vi "json.generate_object.vi"(8 "error in":errorcluster, 11 "ts.iso8601 in":refnum<class "ts.iso8601.lvclass">) -> (0 "error out":errorcluster, 2 "JSON Object":string, 3 "ts.iso8601 out":refnum<class "ts.iso8601.lvclass">)   [LabVIEW 2020, in "ts.iso8601.lvclass"]
uses:
  ts.iso8601.lvclass
  C:/code/labview-client/lv_src/timestampMetadata/timestampMetadata.lvclass
  timestampMetadata/timestampMetadata.lvclass/timestampMetadata.ctl
  fc4585b6-f5f8-418e-b4b0-6256cccee070.vi
  timestampMetadata/seriesName.get.vi
  <vilib>/JDP Science/JSONtext/Variant to JSON Text.vi
  <vilib>/JDP Science/JSONtext/LVClass Serializer/JSONtext LVClass Serializer.lvclass
  ts.iso8601.lvclass/ts.iso8601.ctl
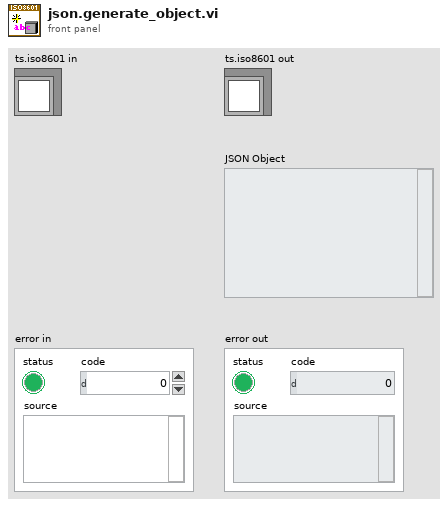
[diagram p1: front panel]
types:
  T1 = cluster{"seriesName":string, "timestampType":cluster{"type":string, "absolute":cluster{"type":string}}}
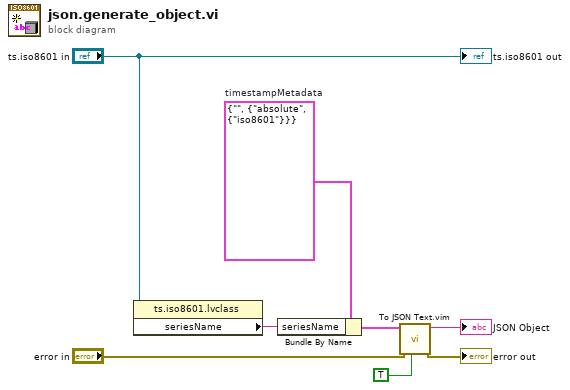
[diagram p0: block diagram]
diagram:
  w1 = T1 {"seriesName"="", "timestampType"={"type"="absolute", "absolute"={"type"="iso8601"}}}  # timestampMetadata
  n1 = property class="ts.iso8601.lvclass"(reference="ts.iso8601 in") -> ("seriesName"=w8:string)  [unwired: 1 in, 2 out]
  n2 = Bundle By Name(cluster=w1, "seriesName"=w8) -> (w7:T1)
  n3 = call "To JSON Text.vim"("Pretty Print?"=TRUE, "error in (no error)"="error in", "Anything"=w7) -> ("error out"=→"error out":errorcluster, "<JSON>"=→"JSON Object":string)  [unwired: 7 in]
  "ts.iso8601 out" <- "ts.iso8601 in"
